vi "UPPER CASE while typing.vi"() -> ()   [LabVIEW 2018]
panel:
  in  "stop":bool
  out "all upper case string":string
  in  "String":string
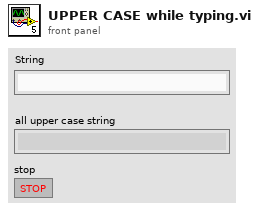
[diagram p1: front panel]
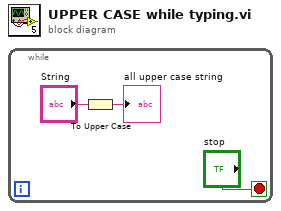
[diagram p0: block diagram]
diagram:
  n1 = while {
    stop <- "stop" stop-if-true
    n2 = To Upper Case(1:"String") -> (0:→"all upper case string":string)
  }
